vi "delete-getTrigger.vi"(8 "error in (no error)":errorcluster, 11 "Instrument.Lockin":refnum<class "Instrument.Lockin.lvclass">) -> (0 "error out":errorcluster, 2 "Trigger":bool, 3 "Instrument.Lockin":refnum<class "Instrument.Lockin.lvclass">)   [LabVIEW 2019, in "Instrument.Lockin.lvclass"]
doc: "API to get the results of lockin calculation.\n\nIf address=\"\", this API reads from localhost\nIf address is remote lockin, you need to add this computer to allowed whitelist on the lockin computer you are trying to access."
uses:
  Instrument.Lockin.lvclass
  Typedefs/API/Lockin.Commands--Enum.ctl
  7e544eb3-996b-42a4-bc58-9c2ab52d037d.vi
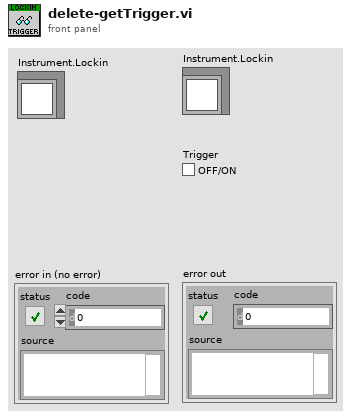
[diagram p1: front panel]
types:
  T1 = typedef "Instrument.Lockin.lvclass/Lockin.Commands--Enum.ctl" = enum16{"setAO", "setAO_Amplitude", "setAO_DC", "setAO_Frequency", "setAO_Phase", "setAO_Function", "setAO_I+", "setREF", "setREF_Frequency", "setREF_Phase", "setREF_TC", "setREF_Roll-Off", "setIVmode", "setDAQ", "Reset", "setSampling", "setOffset", "Trigger", "getAO", "getAI", "getResults", "getTrigger", "getIVmode", "getSampling", "getAOconfig", "getREFconfig", "setInputGain", "setOutputGain", "getInputGain", "getOutputGain", "setAutoSampling", "getAutoSampling", "setSweep", "getStatus", "getSweepResults", "getSweepWaveforms", "startSweep", "stopSweep", "setAUX", "getAUX", "getRefreshTime"}
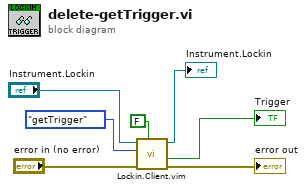
[diagram p0: block diagram]
diagram:
  n1 = call "Lockin.Client.vim"("Data Out type"=FALSE ("setTrigger"), "error in (no error)"="error in (no error)", "Command"=Lockin.Commands--Enum."getTrigger", "Instrument.Lockin in"="Instrument.Lockin") -> ("error out"=→"error out":errorcluster, "Data out"=→"Trigger":bool, "Instrument.Lockin out"=→"Instrument.Lockin":refnum<class "Instrument.Lockin.lvclass">)  [unwired: 5 in]
